vi "Ctor.vi"(8 "error in (no error)":errorcluster, 11 "VISA Client in":refnum<class "Serial Client.lvclass">) -> (0 "error out":errorcluster, 3 "VISA Client out":refnum<class "Serial Client.lvclass">)   [LabVIEW 2020, in "Stream-Serial.lvlib" / "Serial Client.lvclass"]
doc: "Initializes a new client instance that will be ready to configure before opening the connection. Unless using <b>Configure Serial Stream</b>, this VI must be called before calling any of the other VIs in this class or parent classes."
uses:
  Serial Client.lvclass
  Client Command.ctl
  Ref Data.ctl
  Serial Stream/Serial Stream.lvclass
  Port Config.ctl
  Stop Bits.ctl
  Flow Control.ctl
  Parity.ctl
  Serial Client.lvclass/Serial Client.ctl
  <vilib>/IlluminatedG/lv-stream/Connection/Connection.lvclass
  Stream-Serial.lvlib
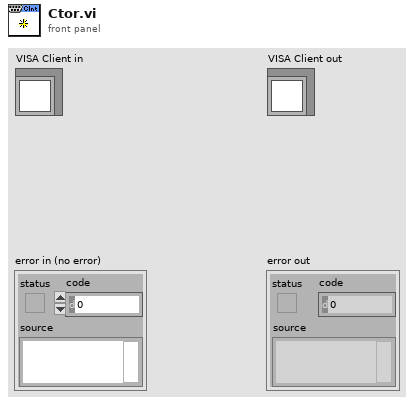
[diagram p1: front panel]
types:
  T1 = typedef "Stream-Serial.lvlib/Serial Client.lvclass/Ref Data.ctl" = cluster{"Stream":refnum<class "Serial Stream.lvclass">, "Client Loop":refnum<vi>, "Port Config":T2, "VISA Resource":refnum<visa-resource-name>}
  T2 = typedef "Stream-Serial.lvlib/Serial Client.lvclass/Port Config.ctl" = cluster{"Baud (115200)":u32, "Data Bits (8)":u8, "Stop Bits (1)":T3, "Flow Control":T4, "Use LineTerm?":bool, "LineTerm (\\n)":string, "Timeout ms (10000)":i32, "Parity (None)":T5}
  T3 = typedef "Stream-Serial.lvlib/Serial Client.lvclass/Stop Bits.ctl" = u16
  T4 = typedef "Stream-Serial.lvlib/Serial Client.lvclass/Flow Control.ctl" = u16
  T5 = typedef "Stream-Serial.lvlib/Serial Client.lvclass/Parity.ctl" = enum16{"None", "Odd", "Even", "Mark", "Space"}
  T6 = typedef "Stream-Serial.lvlib/Client Command.ctl" = enum16{"Connect", "Close", "Shutdown", "Reconnect"}
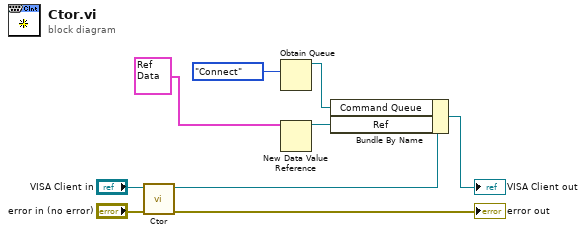
[diagram p0: block diagram]
diagram:
  n1 = call-parent "Ctor.vi"("error in (no error)"="error in (no error)", "Connection in"="VISA Client in") -> ("error out"=→"error out":errorcluster, "Connection out"=w6:refnum<class "Serial Client.lvclass">)  [unwired: 8 in]
  n2 = Obtain Queue(element data type=Client_Command."Connect" ("Command")) -> (queue out=w3:refnum<queue>)  [unwired: 4 in, 2 out]
  n3 = New Data Value Reference(data value=T1 {"Stream"=refnum, "Client Loop"=refnum, "Port Config"={"Baud (115200)"=115200, "Data Bits (8)"=8, "Stop Bits (1)"=10, "Flow Control"=0, "Use LineTerm?"=FALSE, "LineTerm (\\n)"="", "Timeout ms (10000)"=10000, "Parity (None)"=enum."None"}, "VISA Resource"=""} ("Ref Data")) -> (data value reference=w1:refnum<data-value>)  [unwired: 1 in, 1 out]
  n4 = Bundle By Name(cluster=w6, "Command Queue"=w3, "Ref"=w1) -> (→"VISA Client out":refnum<class "Serial Client.lvclass">)
